vi "ncr and npr.vi"() -> ()   [LabVIEW 2024]
panel:
  out "Numeric":dbl
  out "npr":dbl
  in  "r":dbl
  in  "n":dbl
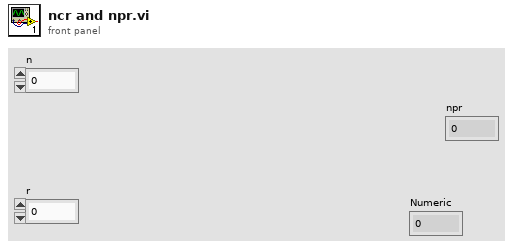
[diagram p1: front panel]
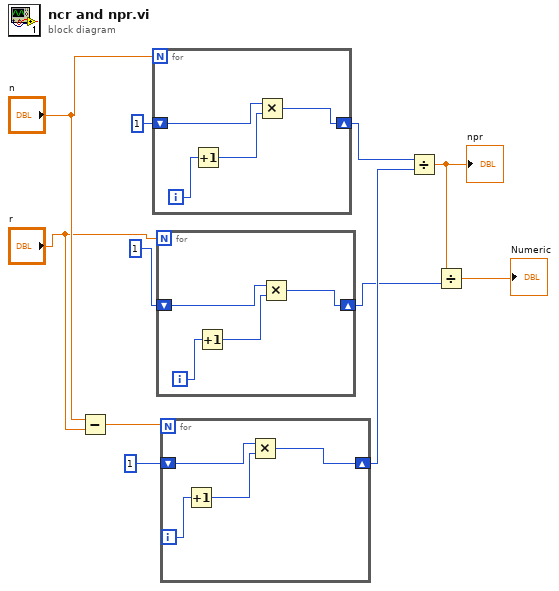
[diagram p0: block diagram]
diagram:
  n1 = Subtract(x="n", y="r") -> (x-y=w6:dbl)
  n2 = for {
    N: "n" -> [_]
    shift-right: [w12] -> w5
    shift-left: 1 -> [w13]
    i -> [w14]
    n3 = Increment(x=w14) -> (x+1=w15:i32)
    n4 = Multiply(x=w13, y=w15) -> (x*y=w12:i32)
  }
  n5 = for {
    N: "r" -> [_]
    shift-right: [w16] -> w3
    shift-left: 1 -> [w17]
    i -> [w18]
    n6 = Increment(x=w18) -> (x+1=w19:i32)
    n7 = Multiply(x=w17, y=w19) -> (x*y=w16:i32)
  }
  n8 = for {
    N: w6 -> [_]
    shift-right: [w20] -> w4
    shift-left: 1 -> [w21]
    i -> [w22]
    n9 = Increment(x=w22) -> (x+1=w23:i32)
    n10 = Multiply(x=w21, y=w23) -> (x*y=w20:i32)
  }
  n11 = Divide(x=w5, y=w4) -> (x/y=w2:dbl)
  "npr" <- w2
  n12 = Divide(x=w2, y=w3) -> (x/y=→"Numeric":dbl)
